vi "Read Camera Status.vi"(8 "error in (no error)":errorcluster, 11 "Interface in":refnum<class "Interface.lvclass">) -> (0 "error out":errorcluster, 2 "Camera Status":T1, 3 "Interface out":refnum<class "Interface.lvclass">)   [LabVIEW 2018, in "Interface.lvclass"]
uses:
  Interface.lvclass
  Interface.lvclass/Interface.ctl
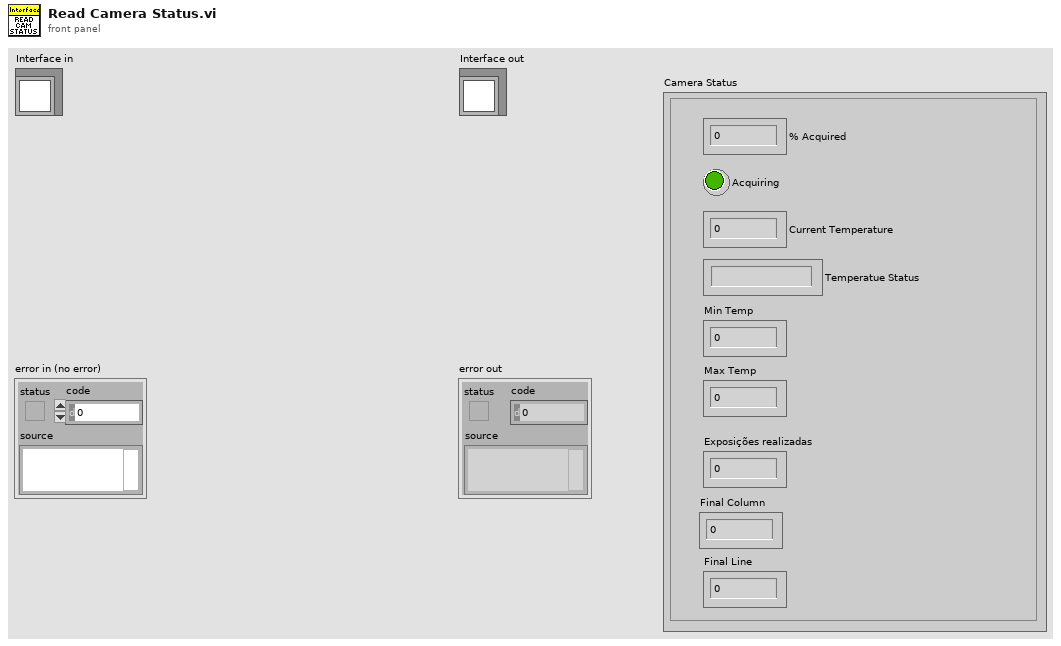
[diagram p1: front panel]
types:
  T1 = cluster{"% Acquired":dbl, "Acquiring":bool, "Current Temperature":dbl, "Temperatue Status":string, "Min Temp":dbl, "Max Temp":dbl, "Exposições realizadas":u32, "Final Column":u16, "Final Line":u16}
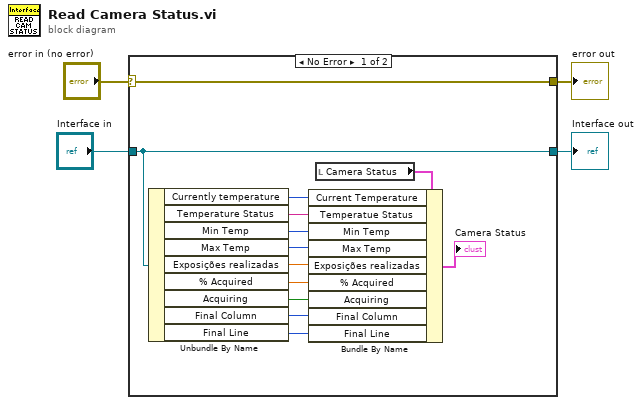
[diagram p0: block diagram]
diagram:
  n1 = case shown="No Error" "error in (no error)" {
    selector: "error in (no error)" -> [w17 w19]
    tunnel: [w17 w19] -> w3
    tunnel: [w14 w18] -> w1
    tunnel: "Interface in" -> [w14 w18]
    frame No Error {
      n2 = Unbundle By Name(w14) -> ("Currently temperature"=w13:i8, "Temperature Status"=w12:string, "Min Temp"=w11:i8, "Max Temp"=w10:i8, "Exposições realizadas"=w9:dbl, "% Acquired"=w7:dbl, "Acquiring"=w8:bool, "Final Column"=w6:u16, "Final Line"=w5:u16)
      n3 = local read "Camera Status"() -> (w15:T1)
      n4 = Bundle By Name(cluster=w15, "Current Temperature"=w13, "Temperatue Status"=w12, "Min Temp"=w11, "Max Temp"=w10, "Exposições realizadas"=w9, "% Acquired"=w7, "Acquiring"=w8, "Final Column"=w6, "Final Line"=w5) -> (→"Camera Status":T1)
    }
    frame Error {
    }
  }
  "error out" <- w3
  "Interface out" <- w1
